vi "LabVIEW Versions Installed Registry.vi"(8 "error in (no error)":errorcluster) -> (0 "error out":errorcluster, 1 "Current Version":T1, 2 "LabVIEW Run-Time Versions":T1[](array[typedef]), 3 "LabVIEW Development Versions":T1[](array[typedef]))   [LabVIEW 2011]
doc: "This VI will return all the versions of LabVIEW installed and the full paths to each version of LabVIEW. It does this through the Windows registry.\n\nReturned on <B>LabVIEW Run-Time Versions</B> will be the versions of the Run-Time engines installed, and <B>LabVIEW Development Versions</B> will have the versions of the development environment that are installed. Both will have similar information, like the version name, as a string or number, and the path to the installed version."
uses:
  <userlib>/_Magna/Application Control/_Controls/magna_e_Type Def - LabVIEW Version Info.ctl
  <vilib>/registry/registry.llb/Registry RtKey.ctl
  <vilib>/registry/registry.llb/Registry SAM.ctl
  <userlib>/_OpenG.lib/array/array.llb/Filter 1D Array with Scalar (String)__ogtk.vi
  <userlib>/_OpenG.lib/array/array.llb/Search 1D Array (Boolean)__ogtk.vi
  <userlib>/_OpenG.lib/array/array.llb/Index 1D Array Elements (String)__ogtk.vi
  <userlib>/_OpenG.lib/array/array.llb/Conditional Auto-Indexing Tunnel (Variant)__ogtk.vi
  <userlib>/_OpenG.lib/array/array.llb/Conditional Auto-Indexing Tunnel (String)__ogtk.vi
  <userlib>/_OpenG.lib/array/array.llb/Search 1D Array (String)__ogtk.vi
  <userlib>/_OpenG.lib/array/array.llb/Delete Elements from Array__ogtk.vi
  <userlib>/_OpenG.lib/array/array.llb/Delete Elements from 1D Array (String)__ogtk.vi
  <userlib>/_OpenG.lib/array/array.llb/Sort Array__ogtk.vi
  <userlib>/_OpenG.lib/array/array.llb/Sort 1D Array (I32)__ogtk.vi
  <userlib>/_OpenG.lib/array/array.llb/Reorder Array2__ogtk.vi
  <userlib>/_OpenG.lib/array/array.llb/Reorder 1D Array2 (String)__ogtk.vi
  <vilib>/registry/registry.llb/Read Registry Value Simple STR.vi
  <vilib>/Utility/config.llb/Read Key (I32).vi
  <vilib>/Utility/config.llb/NI_LVConfig.lvlib
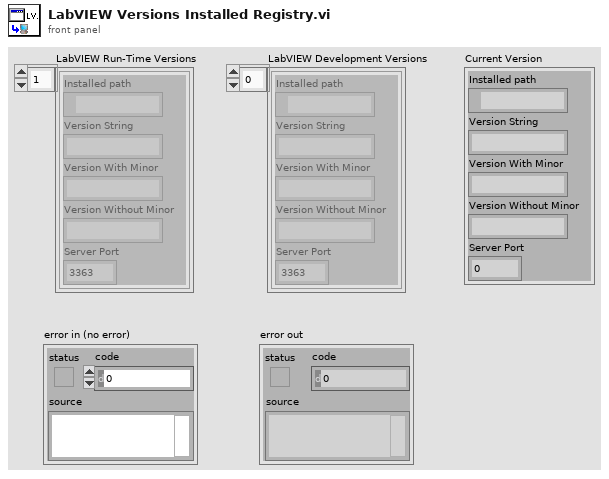
[diagram p1: front panel]
types:
  T1 = typedef "magna_e_Type Def - LabVIEW Version Info.ctl" = cluster{"Installed path":path, "Version String":string, "Version With Minor":string, "Version Without Minor":string, "Server Port":i32}
  T2 = typedef "Registry SAM.ctl" = enum32{"KEY_QUERY_VALUE", "KEY_SET_VALUE", "KEY_CREATE_SUB_KEY", "KEY_ENUMERATE_SUB_KEYS", "KEY_NOTIFY", "KEY_CREATE_LINK", "KEY_READ", "KEY_WRITE", "KEY_ALL_ACCESS", "KEY_READ | KEY_WRITE"}
  T3 = typedef "Registry RtKey.ctl" = enum32{"HKEY_CLASSES_ROOT", "HKEY_CURRENT_USER", "HKEY_LOCAL_MACHINE", "HKEY_USERS", "HKEY_PERFORMANCE_DATA", "HKEY_CURRENT_CONFIG", "HKEY_DYN_DATA"}
  T4 = typedef "Registry refnum.ctl" = refnum<k1>
  T5 = cluster{"numSubKeys":i32, "maxSubKeyLen":i32, "maxSubKeyClassLen":i32}
  T6 = typedef "NI_LVConfig.lvlib/Config Data RefNum.ctl" = refnum<k1>
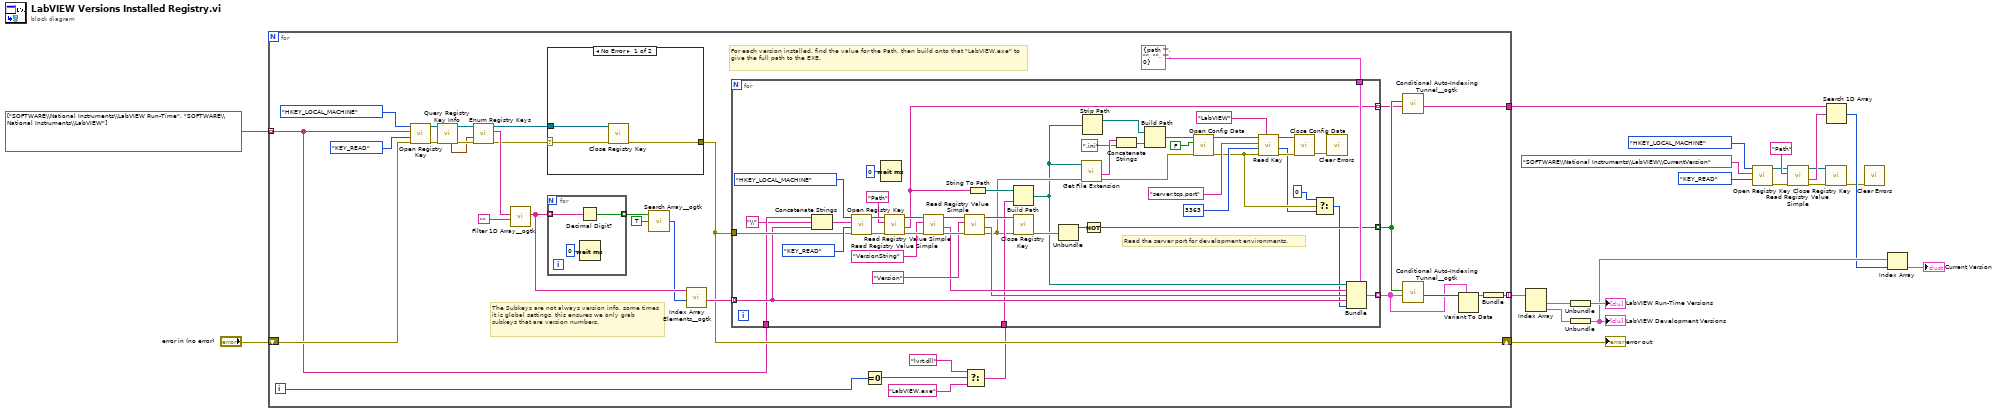
[diagram p0: block diagram]
diagram:
  n1 = for {
    tunnel: string[] ["SOFTWARE\\National Instruments\\LabVIEW Run-Time", "SOFTWARE\\National Instruments\\LabVIEW"] ("subkey") -> [w30] mode=indexing
    shift-right: [w34] -> w19
    shift-left: "error in (no error)" -> [w33]
    tunnel: [w31] -> w18 mode=indexing
    tunnel: [w23] -> w8
    i -> [w29]
    # "For each version installed, find the value for the Path, then build onto that \"LabVIEW.exe\" to give the full path to the EXE."
    # "The Subkeys are not always version info, some times it is global settings, this ensures we only grab subkeys that are version numbers."
    n2 = call <vilib>:"Open Registry Key.vi"("error in (no error)"=w33, "security access mask (KEY_READ | KEY_WRITE)"=Registry_SAM."KEY_READ", "subkey"=w30, "root key (HKEY_LOCAL_MACHINE)"=Registry_RtKey."HKEY_LOCAL_MACHINE") -> ("error out"=w51:errorcluster, "refnum out"=w52:T4)  [unwired: 6 out]
    n3 = call <vilib>:"Query Registry Key Info.vi"("error in (no error)"=w51, "refnum"=w52) -> ("error out"=w49:errorcluster, "refnum out"=w50:T4, "subkey info"=w39:T5)  [unwired: 7 out]
    n4 = call <vilib>:"Enum Registry Keys.vi"("error in (no error)"=w49, "subkey info"=w39, "refnum"=w50) -> ("error out"=w38:errorcluster, "subkeys"=w48:string[], "refnum out"=w41:T4)  [unwired: 6 out]
    n5 = call-poly <userlib>:"Filter 1D Array__ogtk.vi"("items to filter"="", "array"=w48) -> ("filtered array"=w44:string[])  [unwired: 5 out]
    n6 = for {
      tunnel: w44 -> [w106] mode=indexing
      tunnel: [w105] -> w46 mode=indexing
      n7 = Decimal Digit?(1:w106) -> (0:w105:bool)
      n8 = Wait (ms)(milliseconds to wait=u32 0) -> ()  [unwired: 1 out]
    }
    n9 = case shown="No Error" w38 {
      selector: w38 -> [w54 _]
      tunnel: w41 -> [w56 _]
      tunnel: [w55 _] -> w34
      frame No Error {
        n10 = call <vilib>:"Close Registry Key.vi"("error in (no error)"=w54, "refnum"=w56) -> ("error out"=w55:errorcluster)  [unwired: 5 out]
      }
      frame Error {
        # "No Versions of LabVIEW are installed."
      }
    }
    n11 = call-poly <userlib>:"Search Array__ogtk.vi"("Array"=w46, "Element Data"=TRUE) -> ("Indices of Elements"=w43:i32[])  [unwired: 1 in, 6 out]
    n12 = call-poly <userlib>:"Index Array Elements__ogtk.vi"("indices"=w43, "array"=w44) -> ("elements"=w42:string[])  [unwired: 9 out]
    n13 = Equal To 0?(x=w29) -> (x = 0?=w28:bool)
    n14 = Select(t="lvrt.dll" ("name or relative path"), s=w28, f="LabVIEW.exe" ("name or relative path")) -> (s? t:f=w25:string)
    n15 = for {
      tunnel: w42 -> [w87] mode=indexing
      tunnel: w34 -> [w97]
      tunnel: [w86] -> w35 mode=indexing
      tunnel: T1 {"Installed path"=path "", "Version String"="", "Version With Minor"="", "Version Without Minor"="", "Server Port"=0} -> [w85]
      tunnel: [w82] -> w24 mode=indexing
      tunnel: w30 -> [w81]
      tunnel: w25 -> [w79]
      tunnel: [w57] -> w22 mode=indexing
      # "Read the server port for development environments."
      n16 = Concatenate Strings(w81, "\\" ("string"), w87) -> (w102:string)
      n17 = call <vilib>:"Open Registry Key.vi"("error in (no error)"=w97, "security access mask (KEY_READ | KEY_WRITE)"=Registry_SAM."KEY_READ", "subkey"=w102, "root key (HKEY_LOCAL_MACHINE)"=Registry_RtKey."HKEY_LOCAL_MACHINE") -> ("error out"=w101:errorcluster, "refnum out"=w100:T4)  [unwired: 6 out]
      n18 = Wait (ms)(milliseconds to wait=u32 0) -> ()  [unwired: 1 out]
      n19 = call-poly <vilib>:"Read Registry Value Simple.vi"("error in (no error)"=w101, "value"="Path", "refnum"=w100) -> ("error out"=w96:errorcluster, "String/Binary data"=w57:string, "refnum out"=w95:T4)  [unwired: 1 in, 3 out]
      n20 = call-poly <vilib>:"Read Registry Value Simple.vi"("error in (no error)"=w96, "value"="VersionString", "refnum"=w95) -> ("error out"=w92:errorcluster, "String/Binary data"=w89:string, "refnum out"=w93:T4)  [unwired: 1 in, 3 out]
      n21 = call-poly <vilib>:"Read Registry Value Simple.vi"("error in (no error)"=w92, "value"="Version", "refnum"=w93) -> ("error out"=w64:errorcluster, "String/Binary data"=w88:string, "refnum out"=w91:T4)  [unwired: 1 in, 3 out]
      n22 = String To Path(string=w57) -> (path=w65:path)
      n23 = Build Path(base path=w65, name or relative path=w79) -> (appended path=w63:path)
      n24 = call <vilib>:"Close Registry Key.vi"("error in (no error)"=w64, "refnum"=w91) -> ("error out"=w84:errorcluster)  [unwired: 5 out]
      n25 = Unbundle(w84) -> ("status"=w83:bool)  [unwired: 2 out]
      n26 = call <vilib>:"Get File Extension.vi"("error in (no error)"=w64, "file"=w63) -> ("error out"=w73:errorcluster, "filename without extension"=w78:string)  [unwired: 6 in, 2 out]
      n27 = Strip Path(path=w63) -> (stripped path=w68:path)  [unwired: 1 out]
      n28 = Not(x=w83) -> (.not. x?=w82:bool)
      n29 = Concatenate Strings(w78, ".ini" ("string")) -> (w67:string)
      n30 = Build Path(base path=w68, name or relative path=w67) -> (appended path=w66:path)
      n31 = call <vilib>:"Open Config Data.vi"("error in (no error)"=w73, "create file if necessary (T)"=FALSE, "configuration file path"=w66) -> ("error out"=w60:errorcluster, "refnum"=w76:T6)  [unwired: 6 in, 1 out]
      n32 = call-poly <vilib>:"Read Key.vi"("section"="LabVIEW", "error in (no error)"=w60, "default value"=3363, "key"="server.tcp.port", "refnum"=w76) -> ("error out"=w74:errorcluster, "value"=w59:i32, "refnum out"=w75:T6)  [unwired: 3 in, 1 out]
      n33 = call <vilib>:"Close Config Data.vi"("error in (no error)"=w74, "refnum"=w75) -> ("error out"=w62:errorcluster)  [unwired: 8 in, 1 out]
      n34 = Select(t=0, s=w60, f=w59) -> (s? t:f=w58:i32)
      n35 = call <vilib>:"Clear Errors.vi"("error in (no error)"=w62) -> ()  [unwired: 6 in, 1 out]
      n36 = Bundle(cluster=w85, "Installed path"=w63, "Version String"=w89, "Version With Minor"=w88, "Version Without Minor"=w87, "Server Port"=w58) -> (w86:T1)
    }
    n37 = call-poly <userlib>:"Conditional Auto-Indexing Tunnel__ogtk.vi"("Array in"=w22, "Elements to keep"=w24) -> ("Filtered Array out"=w23:string[])  [unwired: 5 in]
    n38 = call-poly <userlib>:"Conditional Auto-Indexing Tunnel__ogtk.vi"("Array in"=w35, "Elements to keep"=w24) -> ("Filtered Array out"=w36:variant[])  [unwired: 5 in]
    n39 = Variant To Data(type=w35, Variant=w36) -> (data=w32:T1[])  [unwired: 1 in, 1 out]
    n40 = Bundle(w32) -> (w31:cluster{T1[]})  [unwired: 1 in]
  }
  "error out" <- w19
  n41 = Index Array(array=w18) -> (element #1=w17:cluster{T1[]}, element #2=w16:cluster{T1[]})  [unwired: 2 in]
  n42 = Unbundle(w17) -> (→"LabVIEW Run-Time Versions":T1[])
  n43 = Unbundle(w16) -> (w4:T1[])
  "LabVIEW Development Versions" <- w4
  n44 = call <vilib>:"Open Registry Key.vi"("security access mask (KEY_READ | KEY_WRITE)"=Registry_SAM."KEY_READ", "subkey"="SOFTWARE\\National Instruments\\LabVIEW\\CurrentVersion", "root key (HKEY_LOCAL_MACHINE)"=Registry_RtKey."HKEY_LOCAL_MACHINE") -> ("error out"=w9:errorcluster, "refnum out"=w10:T4)  [unwired: 1 in, 6 out]
  n45 = call-poly <vilib>:"Read Registry Value Simple.vi"("error in (no error)"=w9, "value"="Path", "refnum"=w10) -> ("error out"=w5:errorcluster, "String/Binary data"=w7:string, "refnum out"=w6:T4)  [unwired: 1 in, 3 out]
  n46 = call <vilib>:"Close Registry Key.vi"("error in (no error)"=w5, "refnum"=w6) -> ("error out"=w1:errorcluster)  [unwired: 5 out]
  n47 = Search 1D Array(1D array=w8, element=w7) -> (index of element=w3:i32)  [unwired: 1 in]
  n48 = call <vilib>:"Clear Errors.vi"("error in (no error)"=w1) -> ()  [unwired: 6 in, 1 out]
  n49 = Index Array(array=w4, index=w3) -> (element=→"Current Version":T1)
